vi "GUI_V_1.vi"() -> ()   [LabVIEW 2014]
uses:
  Users/anjan/Documents/LabVIEW Data/GUI_NEW/Control 1.ctl
  Users/anjan/Documents/LabVIEW Data/GUI_NEW/Global 2.vi
  Users/anjan/Documents/LabVIEW Data/GUI_NEW/Global 1.vi
panel:
  in  "Acc Alarm Setpoint":i32
  out "Acc Alarm":bool
  out "IR Alarm":bool
  in  "IR Alarm Setpoint":i32
  in  "Stop":bool
  out "Operation Mode":T1
  in  "Fall Detect Mode":bool
  in  "IR Mode":bool
  out "IR Data Measurement":dbl(graph)
  out "Accelerometer Data Measurement":dbl(graph)
  # "MOBILE TRACKING SYSTEM"
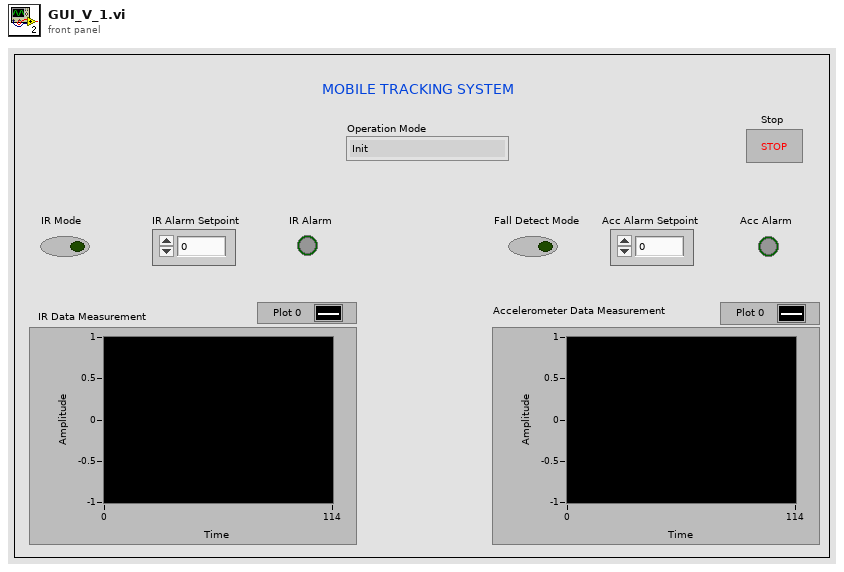
[diagram p1: front panel]
types:
  T1 = typedef "Control 1.ctl" = enum16{"Init", "Select Operation Mode", "IR Selection", "Fall Detect Selection", "Shutdown"}
  T2 = enum8{"Enabled", "Disabled", "Disabled and Grayed Out"}
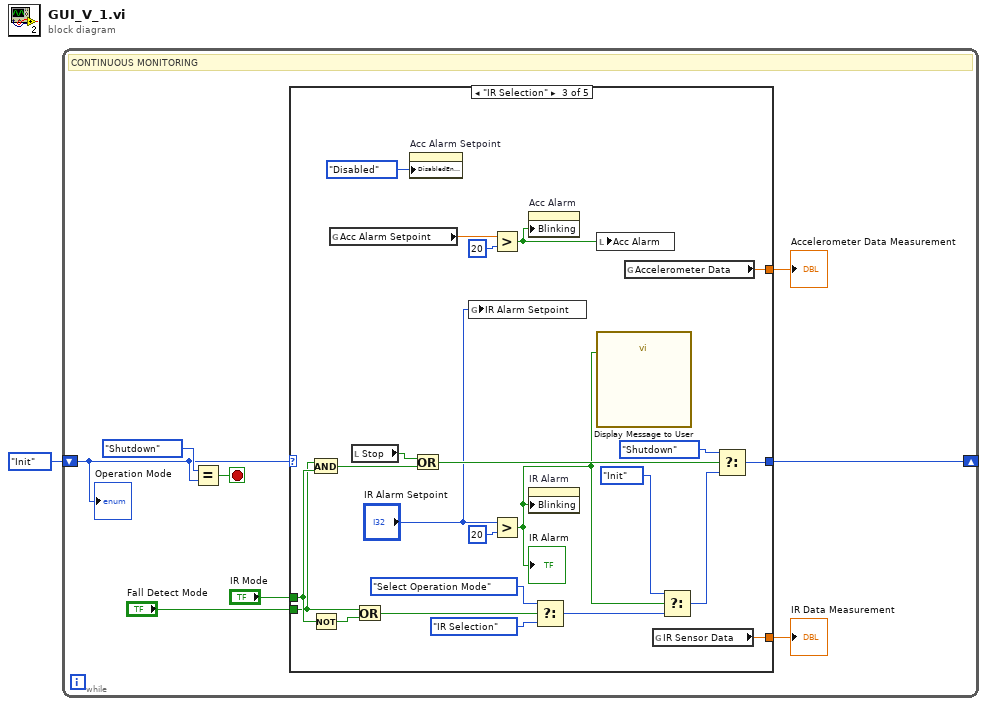
[diagram p0: block diagram]
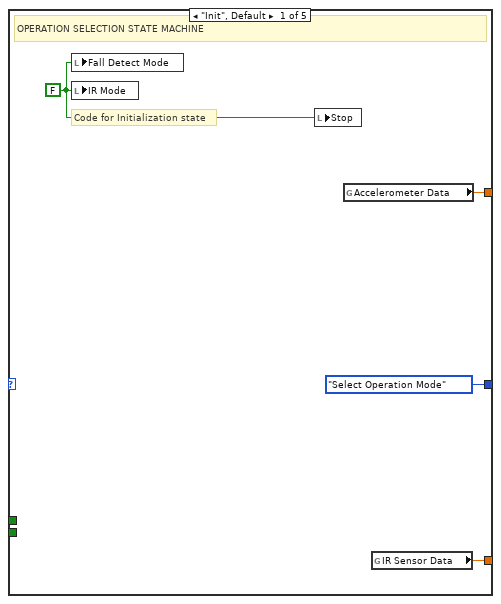
[diagram p2: hidden frame]
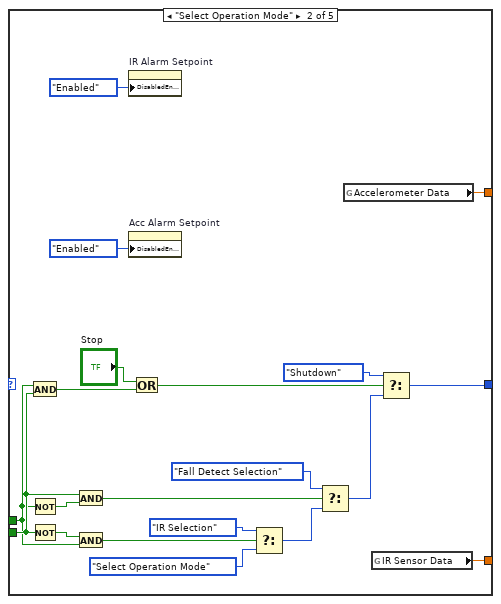
[diagram p3: hidden frame]
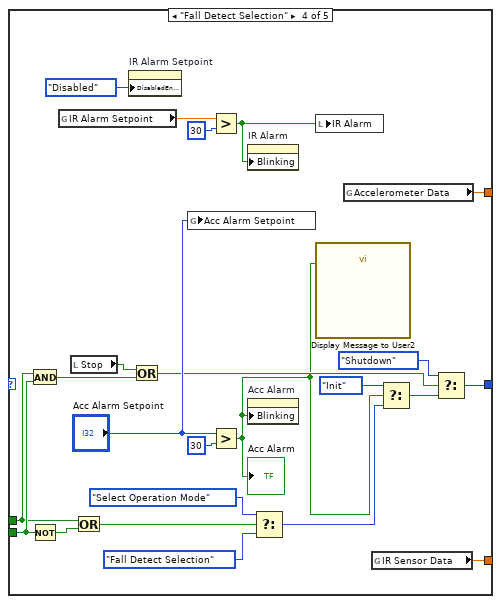
[diagram p4: hidden frame]
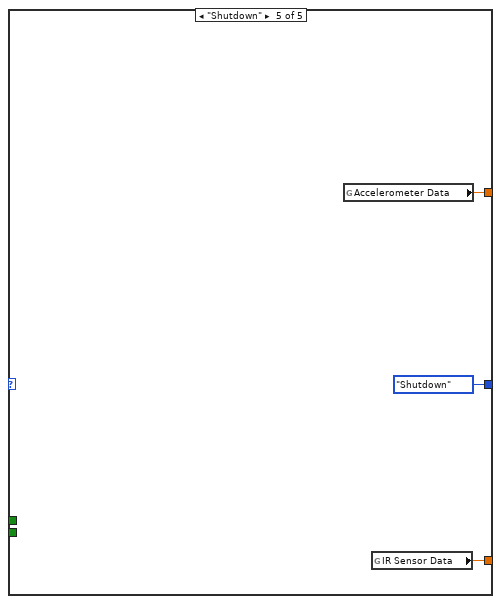
[diagram p5: hidden frame]
diagram:
  n1 = while {
    shift-right: [w9] -> _
    shift-left: Control_1."Init" ("Operation Mode") -> [w6]
    stop <- w8 stop-if-true
    # "CONTINUOUS MONITORING"
    n2 = Equal?(x=Control_1."Shutdown" ("Operation Mode"), y=w6) -> (x = y?=w8:bool)
    n3 = case shown="\"IR Selection\"" w6 {
      tunnel: [Control_1."Select Operation Mode" ("Operation Mode") w30 w53 w74 Control_1."Shutdown" ("Operation Mode")] -> w9
      tunnel: "Fall Detect Mode" -> [_ w19 w43 w64 _]
      tunnel: "IR Mode" -> [_ w18 w44 w63 _]
      tunnel: [w10 w17 w42 w61 w80] -> w3
      tunnel: [w11 w16 w41 w62 w81] -> w2
      frame "Init", Default {
        w12 = FALSE ("stop")
        # "Code for Initialization state"
        # "OPERATION SELECTION STATE MACHINE"
        n4 = local write "Fall Detect Mode"(w12) -> ()
        n5 = local write "IR Mode"(w12) -> ()
        n6 = local write "Stop"(w12) -> ()
        n7 = global read "Global 2.vi" "Accelerometer Data"() -> (w11:dbl)
        n8 = global read "Global 2.vi" "IR Sensor Data"() -> (w10:dbl)
      }
      frame "Select Operation Mode" {
        n9 = And(x=w18, y=w19) -> (x .and. y?=w21:bool)
        n10 = Not(x=w18) -> (.not. x?=w24:bool)
        n11 = Not(x=w19) -> (.not. x?=w23:bool)
        n12 = And(x=w19, y=w24) -> (x .and. y?=w25:bool)
        n13 = And(x=w23, y=w18) -> (x .and. y?=w26:bool)
        n14 = property on="IR Alarm Setpoint" class="DigNum (strict)"("DisabledEnum"=T2."Enabled" ("Disabled")) -> ()  [unwired: 2 in, 2 out]
        n15 = property on="Acc Alarm Setpoint" class="DigNum (strict)"("DisabledEnum"=T2."Enabled" ("Disabled")) -> ()  [unwired: 2 in, 2 out]
        n16 = Or(x="Stop", y=w21) -> (x .or. y?=w20:bool)
        n17 = Select(t=Control_1."IR Selection" ("Operation Mode"), s=w26, f=Control_1."Select Operation Mode" ("Operation Mode")) -> (s? t:f=w29:T1)
        n18 = Select(t=Control_1."Fall Detect Selection" ("Operation Mode"), s=w25, f=w29) -> (s? t:f=w28:T1)
        n19 = global read "Global 2.vi" "Accelerometer Data"() -> (w16:dbl)
        n20 = global read "Global 2.vi" "IR Sensor Data"() -> (w17:dbl)
        n21 = Select(t=Control_1."Shutdown" ("Operation Mode"), s=w20, f=w28) -> (s? t:f=w30:T1)
      }
      frame "IR Selection" {
        n22 = And(x=w43, y=w44) -> (x .and. y?=w51:bool)
        n23 = Not(x=w44) -> (.not. x?=w49:bool)
        n24 = global read "Global 1.vi" "Acc Alarm Setpoint"() -> (w34:dbl)
        n25 = local read "Stop"() -> (w52:bool)
        n26 = Or(x=w43, y=w49) -> (x .or. y?=w48:bool)
        n27 = property on="Acc Alarm Setpoint" class="DigNum (strict)"("DisabledEnum"=T2."Disabled" ("Disabled")) -> ()  [unwired: 2 in, 2 out]
        n28 = Or(x=w52, y=w51) -> (x .or. y?=w50:bool)
        n29 = global write "Global 1.vi" "IR Alarm Setpoint"("IR Alarm Setpoint") -> ()
        n30 = Greater?(x=w34, y=20) -> (0:w36:bool)
        n31 = Greater?(x="IR Alarm Setpoint", y=20) -> (0:w39:bool)
        "IR Alarm" <- w39
        n32 = property on="Acc Alarm" class="Bool (strict)"("Blinking"=w36) -> ()  [unwired: 2 in, 2 out]
        n33 = property on="IR Alarm" class="Bool (strict)"("Blinking"=w39) -> ()  [unwired: 2 in, 2 out]
        n34 = Select(t=Control_1."Select Operation Mode" ("Operation Mode"), s=w48, f=Control_1."IR Selection" ("Operation Mode")) -> (s? t:f=w47:T1)
        n35 = local write "Acc Alarm"(w36) -> ()
        n36 = call "Display Message to User"("Enable"=w39) -> ()  [unwired: 9 in, 2 out]
        n37 = global read "Global 2.vi" "Accelerometer Data"() -> (w41:dbl)
        n38 = global read "Global 2.vi" "IR Sensor Data"() -> (w42:dbl)
        n39 = Select(t=Control_1."Init" ("Operation Mode"), s=w39, f=w47) -> (s? t:f=w46:T1)
        n40 = Select(t=Control_1."Shutdown" ("Operation Mode"), s=w50, f=w46) -> (s? t:f=w53:T1)
      }
      frame "Fall Detect Selection" {
        n41 = And(x=w63, y=w64) -> (x .and. y?=w73:bool)
        n42 = Not(x=w64) -> (.not. x?=w70:bool)
        n43 = global read "Global 1.vi" "IR Alarm Setpoint"() -> (w57:dbl)
        n44 = local read "Stop"() -> (w72:bool)
        n45 = Or(x=w63, y=w70) -> (x .or. y?=w69:bool)
        n46 = property on="IR Alarm Setpoint" class="DigNum (strict)"("DisabledEnum"=T2."Disabled" ("Disabled")) -> ()  [unwired: 2 in, 2 out]
        n47 = Or(x=w72, y=w73) -> (x .or. y?=w71:bool)
        n48 = global write "Global 1.vi" "Acc Alarm Setpoint"("Acc Alarm Setpoint") -> ()
        n49 = Greater?(x=w57, y=30) -> (0:w59:bool)
        n50 = Greater?(x="Acc Alarm Setpoint", y=30) -> (0:w65:bool)
        "Acc Alarm" <- w65
        n51 = property on="IR Alarm" class="Bool (strict)"("Blinking"=w59) -> ()  [unwired: 2 in, 2 out]
        n52 = property on="Acc Alarm" class="Bool (strict)"("Blinking"=w65) -> ()  [unwired: 2 in, 2 out]
        n53 = Select(t=Control_1."Select Operation Mode" ("Operation Mode"), s=w69, f=Control_1."Fall Detect Selection" ("Operation Mode")) -> (s? t:f=w67:T1)
        n54 = local write "IR Alarm"(w59) -> ()
        n55 = call "Display Message to User2"("Enable"=w65) -> ()  [unwired: 9 in, 2 out]
        n56 = global read "Global 2.vi" "Accelerometer Data"() -> (w62:dbl)
        n57 = global read "Global 2.vi" "IR Sensor Data"() -> (w61:dbl)
        n58 = Select(t=Control_1."Init" ("Operation Mode"), s=w65, f=w67) -> (s? t:f=w68:T1)
        n59 = Select(t=Control_1."Shutdown" ("Operation Mode"), s=w71, f=w68) -> (s? t:f=w74:T1)
      }
      frame "Shutdown" {
        n60 = global read "Global 2.vi" "Accelerometer Data"() -> (w81:dbl)
        n61 = global read "Global 2.vi" "IR Sensor Data"() -> (w80:dbl)
      }
    }
    "IR Data Measurement" <- w3
    "Accelerometer Data Measurement" <- w2
    "Operation Mode" <- w6
  }
